vi "MatrixVg_Tdep.vi"(0 "T-table String":string, 3 "Time Stamp":timestamp, 6 "Play Button":bool, 7 "Custom Folder":string, 8 "Settings":T3={"Ring 3"=1, "Ring 2"=4, "Fixed Current mkA"=0.5, "If yes, the current is:"=enum."Radio Selection 1", "Ressitance measurements?"=TRUE, "Commute DC current?"=FALSE} {"Ring 3" items=["1 kOhm", "10 kOhm", "100 kOhm", "1 Mohm", "10 mOhm"]; "Ring 2" items=["1 kOhm", "10 kOhm", "100 kOhm", "1 Mohm", "10 MOhm"]}, 9 "Instruments":T4={"Oscillator"=TRUE, "Addr 1 lock-in"=TRUE, "Addr 1 lock-in oop"=TRUE, "Addr 2 lock-in"=TRUE, "Addr 2 lock-in oop"=TRUE, "Addr 3 lock-in"=FALSE, "Addr 3 lock-in oop"=FALSE, "Voltage (Vk1)"=FALSE, "Current (Ik1)"=TRUE, "Voltage (Vk2)"=FALSE, "Current (Ik2)"=FALSE, "Voltage (Vk3)"=FALSE, "Current (Ik3)"=FALSE, "Channel 1 (Vnano1)  "=FALSE, "Channel 2 (Vnano1b)"=FALSE, "Channel 1 (Vnano2)   "=FALSE, "Channel 2 (Vnano2b)"=FALSE, "Thermometer 1 (T1)"=TRUE, "Magnetic Field (B)"=TRUE, "Capacitance (C) and Loss (L)"=FALSE}, 11 "TCluster":T2={"Starting T (K)"=-1.0, "Final T (K)"=1.0, "Step (T)"=1.0, "Stabillisation, min"=1.0, "Wait 1st point?"=FALSE} {"Final T (K)" min=-4.0 max=4.0 step=0.1 format="%.2f"; "Stabillisation, min" format="%.2f"; "Step (T)" min=0.0 max=1.0 step=0.01 format="%_4f"; "Starting T (K)" min=-4.0 max=4.0 step=0.1 format="%.2f"}) -> ()   [LabVIEW 2017]
uses:
  <vilib>/Utility/file.llb/Read From Spreadsheet File (DBL).vi
panel:
  in  "VgCluster":T1={"V1 (V)"=-1.0, "V2 (V)"=1.0, "Sweep rate, V/min"=1.0, "Time btw \npoints, sec"=1.0, "points at each Vg"=1, "Compliance, mkA"=0.05, "No-record rate, V/min"=30.0, "Full sweep?"=FALSE} {"No-record rate, V/min" min=0.0 max=1.0 step=0.01 format="%_4f"; "V2 (V)" min=-4.0 max=4.0 step=0.1 format="%.2f"; "Compliance, mkA" min=0.0 max=1.0 step=0.01 format="%.3f"; "Time btw \npoints, sec" format="%.2f"; "Sweep rate, V/min" min=0.0 max=1.0 step=0.01 format="%_4f"; "V1 (V)" min=-4.0 max=4.0 step=0.1 format="%.2f"}
  out "Communication":string
  out "T Array":dbl[](array[numeric])
  out "Experiment ends at:":string
  out "Hours":dbl format="%.1f"
  out "Estimated time of experiment:":i16
  out "ArraySens":i8[](array[numeric])
  out "ArrayOsc":dbl[](array[numeric])
  out "# of configurations":i8
  out "Large Array":bool[][][](array[boolean])
  out "Contact configuration file (*.conf)":path
  # "hours"
  # "min.="
  # "Values of T can be also entered as the table by copying\nand pasting a column of numbers in a \"T table\" string at the \nfar right side of this window."
  # "Lock-in Amplifiers"
  # "Temperature"
  # "SourceMeters"
  # "Nanovoltmeters"
  # "Main"
  # "(not recommended, too slow)"
  # "Magnetic Field"
  # "Capacitance & Loss"
  # "(not recommended, too slow)"
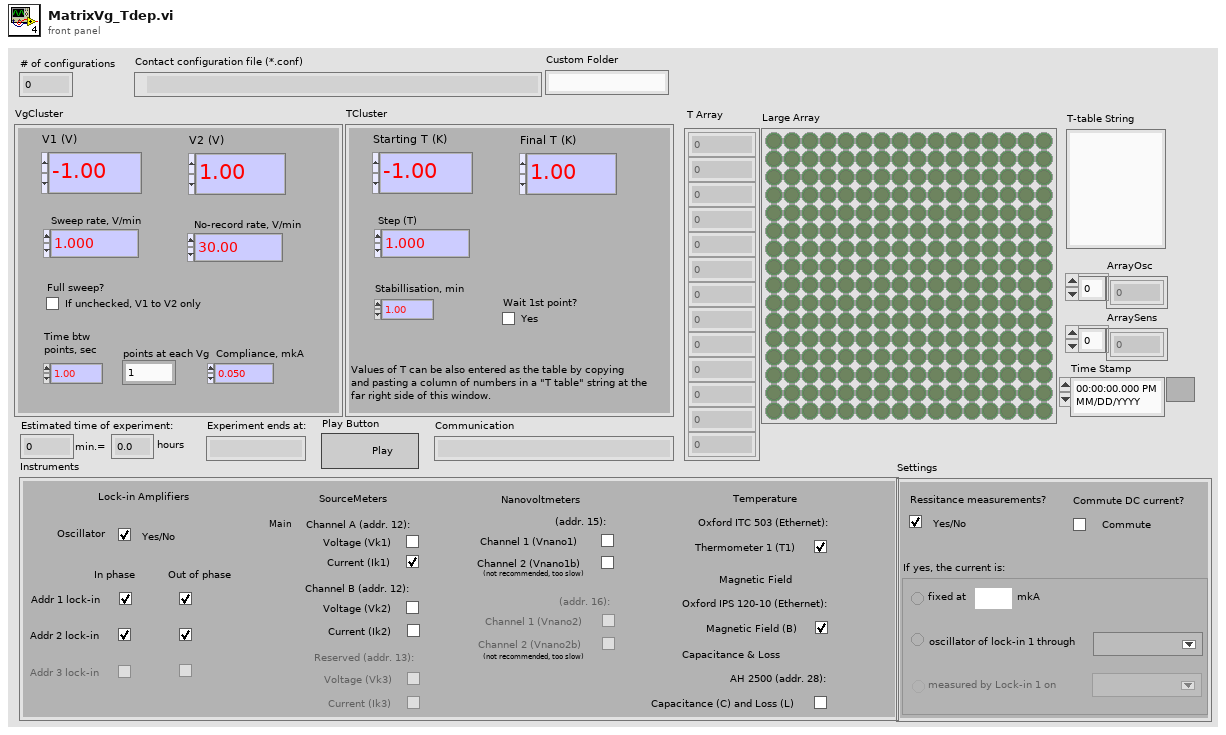
[diagram p1: front panel]
types:
  T1 = cluster{"V1 (V)":dbl, "V2 (V)":dbl, "Sweep rate, V/min":dbl, "Time btw \npoints, sec":dbl, "points at each Vg":i32, "Compliance, mkA":dbl, "No-record rate, V/min":dbl, "Full sweep?":bool}
  T2 = cluster{"Starting T (K)":dbl, "Final T (K)":dbl, "Step (T)":dbl, "Stabillisation, min":dbl, "Wait 1st point?":bool}
  T3 = cluster{"Ring 3":u16, "Ring 2":u16, "Fixed Current mkA":dbl, "If yes, the current is:":enum32{"Radio Selection 1", "Radio Selection 2", "Radio Selection 3"}, "Ressitance measurements?":bool, "Commute DC current?":bool}
  T4 = cluster{"Oscillator":bool, "Addr 1 lock-in":bool, "Addr 1 lock-in oop":bool, "Addr 2 lock-in":bool, "Addr 2 lock-in oop":bool, "Addr 3 lock-in":bool, "Addr 3 lock-in oop":bool, "Voltage (Vk1)":bool, "Current (Ik1)":bool, "Voltage (Vk2)":bool, "Current (Ik2)":bool, "Voltage (Vk3)":bool, "Current (Ik3)":bool, "Channel 1 (Vnano1)  ":bool, "Channel 2 (Vnano1b)":bool, "Channel 1 (Vnano2)   ":bool, "Channel 2 (Vnano2b)":bool, "Thermometer 1 (T1)":bool, "Magnetic Field (B)":bool, "Capacitance (C) and Loss (L)":bool}
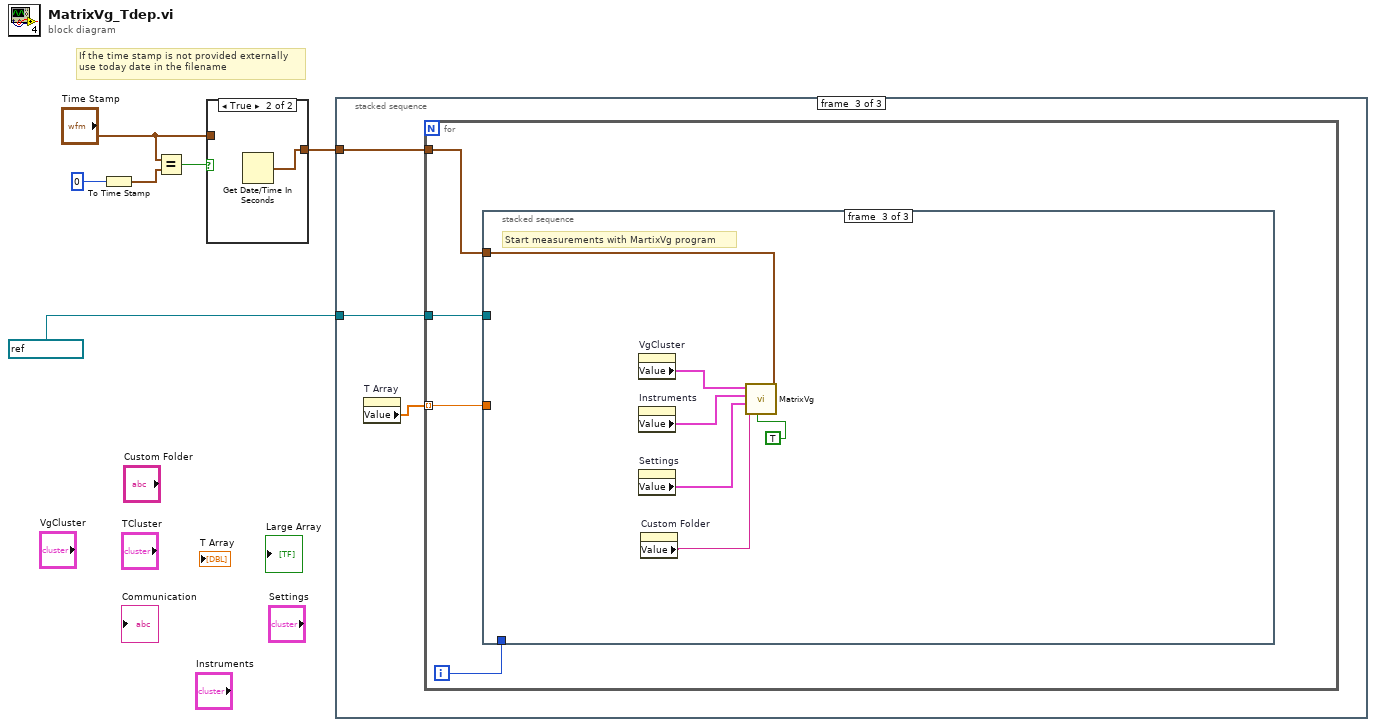
[diagram p0: block diagram]
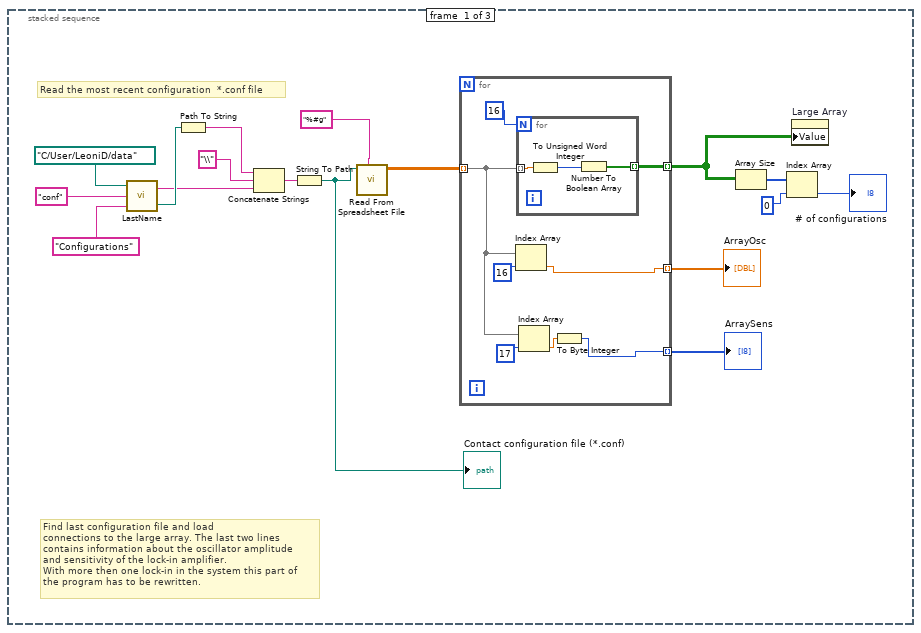
[diagram p3: hidden frame]
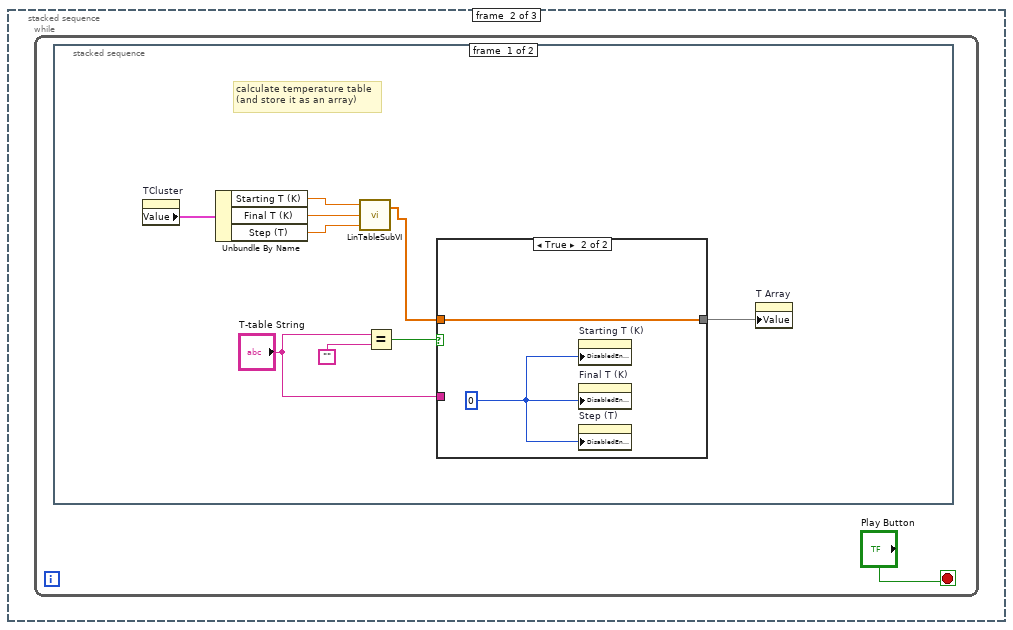
[diagram p4: hidden frame]
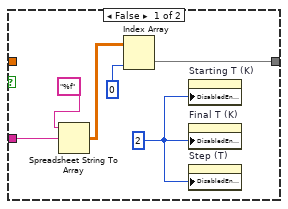
[diagram p5: hidden frame]
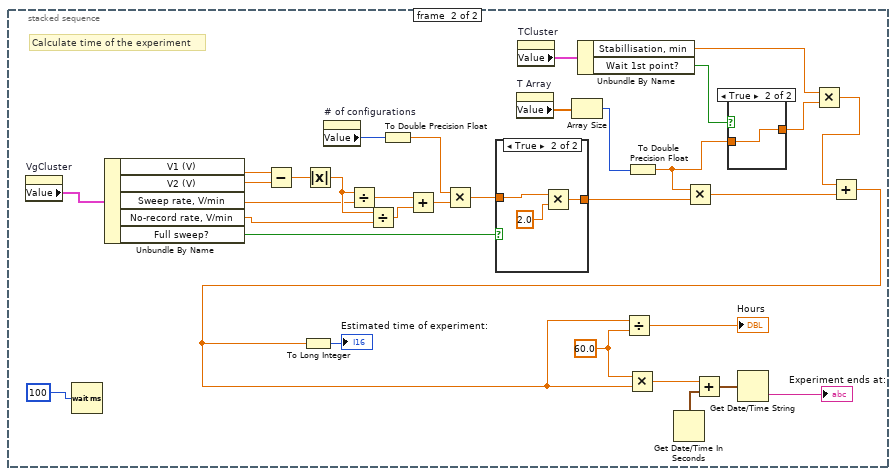
[diagram p6: hidden frame]
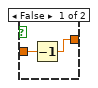
[diagram p7: hidden frame]
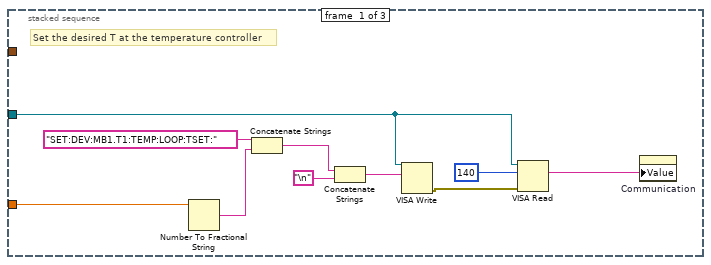
[diagram p9: hidden frame]
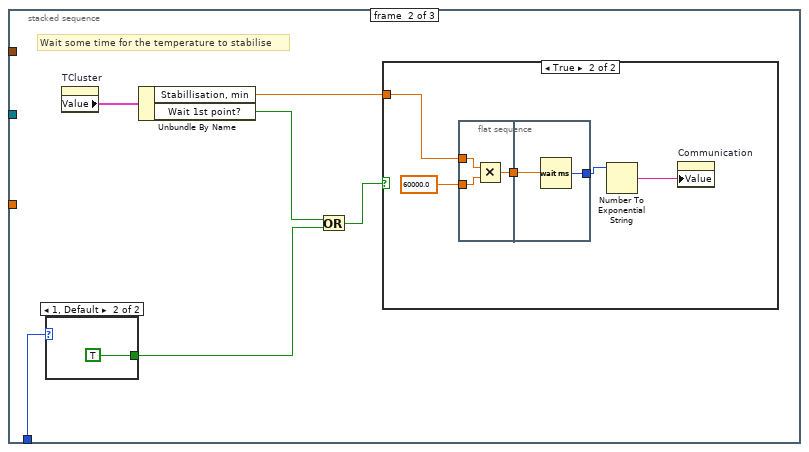
[diagram p10: hidden frame]
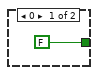
[diagram p12: hidden frame]
diagram:
  # "If the time stamp is not provided externally\nuse today date in the filename"
  n1 = To Time Stamp(1:0) -> (0:w5:timestamp)
  n2 = Equal?(x="Time Stamp", y=w5) -> (x = y?=w4:bool)
  n3 = case shown="True" w4 {
    tunnel: "Time Stamp" -> [w7 _]
    tunnel: [w7 w8] -> w2
    frame False {
    }
    frame True {
      n4 = Get Date/Time In Seconds() -> (seconds since 1Jan1904=w8:timestamp)
    }
  }
  n5 = stacked-sequence {
    tunnel: w2 -> [_ _ w95]
    tunnel: refnum<visa-resource-name> "itcetherT" ("VISA resource name") -> [_ _ w97]
    frame #0 {
      # "Read the most recent configuration  *.conf file"
      # "Find last configuration file and load \nconnections to the large array. The last two lines \ncontains information about the oscillator amplitude\nand sensitivity of the lock-in amplifier.\nWith more then one lock-in in the system this part of \nthe program has to be rewritten."
      n6 = call "LastName.vi"("Custom Folder"="Configurations", "Extention"="conf", "User Data Folder"=path "C:/User/LeoniD/data") -> ("created path"=w21:path, "String"=w20:string)
      n7 = Path To String(path=w21) -> (string=w25:string)
      n8 = Concatenate Strings(w25, "\\", w20) -> (w23:string)
      n9 = String To Path(string=w23) -> (path=w11:path)
      "Contact configuration file (*.conf)" <- w11
      n10 = call-poly <vilib>:"Read From Spreadsheet File.vi"("format (%.3f)"="%#g", "file path (dialog if empty)"=w11) -> ("all rows"=w16:dbl[][])  [unwired: 5 in, 4 out]
      n11 = for {
        tunnel: w16 -> [w29] mode=indexing
        tunnel: [w33] -> w13 mode=indexing
        tunnel: [w28] -> w10 mode=indexing
        tunnel: [w27] -> w9 mode=indexing
        n12 = Index Array(array=w29, index=16) -> (element=w28:dbl)
        n13 = for {
          N: 16 -> [_]
          tunnel: w29 -> [w36] mode=indexing
          tunnel: [w34] -> w33 mode=indexing
          n14 = To Unsigned Word Integer(number=w36) -> (unsigned 16bit integer=w35:u16)
          n15 = Number To Boolean Array(number=w35) -> (Boolean array=w34:bool[])
        }
        n16 = Index Array(array=w29, index=17) -> (element=w30:dbl)
        n17 = To Byte Integer(number=w30) -> (8bit integer=w27:i8)
      }
      "ArrayOsc" <- w10
      "ArraySens" <- w9
      n18 = Array Size(array=w13) -> (size(s)=w15:i32[])
      n19 = Index Array(array=w15, index=0) -> (element=→"# of configurations":i32)
      n20 = property on="Large Array" class="Arr (strict)"("Value"=w13) -> ()  [unwired: 2 in, 2 out]
    }
    frame #1 {
      n21 = while {
        stop <- "Play Button" stop-if-true
        n22 = stacked-sequence {
          frame #0 {
            # "calculate temperature table\n(and store it as an array)"
            n23 = property on="TCluster" class="Clust (strict)"() -> ("Value"=w42:T2)  [unwired: 2 in, 2 out]
            n24 = Unbundle By Name(w42) -> ("Starting T (K)"=w41:dbl, "Final T (K)"=w40:dbl, "Step (T)"=w39:dbl)
            n25 = call "LinTableSubVI.vi"("Step"=w39, "Final"=w40, "Initial"=w41) -> ("Array"=w46:dbl[])  [unwired: 1 in]
            n26 = Equal?(x="T-table String", y="") -> (x = y?=w43:bool)
            n27 = case shown="True" w43 {
              tunnel: [w49 w54] -> w38
              tunnel: w46 -> [_ w54]
              tunnel: "T-table String" -> [w48 _]
              frame False {
                w47 = 2
                n28 = Spreadsheet String To Array(format string="%f", spreadsheet string=w48) -> (array=w51:dbl[][])  [unwired: 2 in]
                n29 = Index Array(array=w51, index (col)=0) -> (element=w49:dbl[])  [unwired: 1 in]
                n30 = property on="Starting T (K)" class="DigNum (strict)"("DisabledEnum"=w47) -> ()  [unwired: 2 in, 2 out]
                n31 = property on="Final T (K)" class="DigNum (strict)"("DisabledEnum"=w47) -> ()  [unwired: 2 in, 2 out]
                n32 = property on="Step (T)" class="DigNum (strict)"("DisabledEnum"=w47) -> ()  [unwired: 2 in, 2 out]
              }
              frame True {
                w53 = 0
                n33 = property on="Starting T (K)" class="DigNum (strict)"("DisabledEnum"=w53) -> ()  [unwired: 2 in, 2 out]
                n34 = property on="Final T (K)" class="DigNum (strict)"("DisabledEnum"=w53) -> ()  [unwired: 2 in, 2 out]
                n35 = property on="Step (T)" class="DigNum (strict)"("DisabledEnum"=w53) -> ()  [unwired: 2 in, 2 out]
              }
            }
            n36 = property on="T Array" class="Arr (strict)"("Value"=w38) -> ()  [unwired: 2 in, 2 out]
          }
          frame #1 {
            w67 = 60.0
            # "Calculate time of the experiment"
            n37 = property on="VgCluster" class="Clust (strict)"() -> ("Value"=w86:T1)  [unwired: 2 in, 2 out]
            n38 = Wait (ms)(milliseconds to wait=100) -> ()  [unwired: 1 out]
            n39 = Unbundle By Name(w86) -> ("V1 (V)"=w85:dbl, "V2 (V)"=w84:dbl, "Sweep rate, V/min"=w81:dbl, "No-record rate, V/min"=w80:dbl, "Full sweep?"=w74:bool)
            n40 = Subtract(x=w85, y=w84) -> (x-y=w83:dbl)
            n41 = Absolute Value(x=w83) -> (abs(x)=w82:dbl)
            n42 = property on="# of configurations" class="DigNum (strict)"() -> ("Value"=w76:i8)  [unwired: 2 in, 2 out]
            n43 = Divide(x=w82, y=w81) -> (x/y=w79:dbl)
            n44 = Divide(x=w82, y=w80) -> (x/y=w78:dbl)
            n45 = To Double Precision Float(number=w76) -> (double precision float=w75:dbl)
            n46 = Add(x=w79, y=w78) -> (x+y=w77:dbl)
            n47 = Multiply(x=w75, y=w77) -> (x*y=w73:dbl)
            n48 = case shown="True" w74 {
              tunnel: w73 -> [w91 w94]
              tunnel: [w91 w92] -> w62
              frame False {
              }
              frame True {
                n49 = Multiply(x=w94, y=2.0) -> (x*y=w92:dbl)
              }
            }
            n50 = property on="T Array" class="Arr (strict)"() -> ("Value"=w65:dbl[])  [unwired: 2 in, 2 out]
            n51 = property on="TCluster" class="Clust (strict)"() -> ("Value"=w64:T2)  [unwired: 2 in, 2 out]
            n52 = Array Size(array=w65) -> (size(s)=w63:i32)
            n53 = Unbundle By Name(w64) -> ("Stabillisation, min"=w59:dbl, "Wait 1st point?"=w61:bool)
            n54 = To Double Precision Float(number=w63) -> (double precision float=w60:dbl)
            n55 = Get Date/Time In Seconds() -> (seconds since 1Jan1904=w71:timestamp)
            n56 = Multiply(x=w60, y=w62) -> (x*y=w57:dbl)
            n57 = case shown="True" w61 {
              tunnel: [w89 w90] -> w58
              tunnel: w60 -> [w88 w90]
              frame False {
                n58 = Decrement(x=w88) -> (x-1=w89:dbl)
              }
              frame True {
              }
            }
            n59 = Multiply(x=w59, y=w58) -> (x*y=w56:dbl)
            n60 = Add(x=w56, y=w57) -> (x+y=w55:dbl)
            n61 = To Long Integer(number=w55) -> (32bit integer=→"Estimated time of experiment:":i32)
            n62 = Divide(x=w55, y=w67) -> (x/y=→"Hours":dbl)
            n63 = Multiply(x=w67, y=w55) -> (x*y=w66:dbl)
            n64 = Add(x=w66, y=w71) -> (x+y=w70:timestamp)
            n65 = Get Date/Time String(seconds (now)=w70) -> (time string=→"Experiment ends at:":string)  [unwired: 2 in, 1 out]
          }
        }
      }
    }
    frame #2 {
      n66 = property on="T Array" class="Arr (strict)"() -> ("Value"=w96:dbl[])  [unwired: 2 in, 2 out]
      n67 = for {
        tunnel: w97 -> [w101]
        tunnel: w96 -> [w100] mode=indexing
        tunnel: w95 -> [w98]
        i -> [w99]
        n68 = stacked-sequence {
          tunnel: w101 -> [w102 _ _]
          tunnel: w100 -> [w103 _ _]
          tunnel: w99 -> [_ w113 _]
          tunnel: w98 -> [_ _ w130]
          frame #0 {
            # "Set the desired T at the temperature controller"
            n69 = Number To Fractional String(number=w103) -> (F-format string=w110:string)  [unwired: 3 in]
            n70 = Concatenate Strings("SET:DEV:MB1.T1:TEMP:LOOP:TSET:" ("string"), w110) -> (w105:string)
            n71 = Concatenate Strings(w105, "\n") -> (w106:string)
            n72 = VISA Write(VISA resource name=w102, write buffer=w106) -> (error out=w109:errorcluster)  [unwired: 1 in, 2 out]
            n73 = VISA Read(VISA resource name=w102, byte count=140, error in (no error)=w109) -> (read buffer=w104:string)  [unwired: 3 out]
            n74 = property on="Communication" class="Str"("Value"=w104) -> ()  [unwired: 2 in, 2 out]
          }
          frame #1 {
            # "Wait some time for the temperature to stabilise"
            n75 = case shown="1, Default" w113 {
              tunnel: [FALSE TRUE] -> w117
              frame 0 {
              }
              frame 1, Default {
              }
            }
            n76 = property on="TCluster" class="Clust (strict)"() -> ("Value"=w115:T2)  [unwired: 2 in, 2 out]
            n77 = Unbundle By Name(w115) -> ("Stabillisation, min"=w112:dbl, "Wait 1st point?"=w114:bool)
            n78 = Or(x=w114, y=w117) -> (x .or. y?=w116:bool)
            n79 = case shown="True" w116 {
              tunnel: w112 -> [_ w121]
              frame False {
              }
              frame True {
                n80 = flat-sequence {
                  tunnel: w121 -> [w125]
                  tunnel: 60000.0 -> [w124]
                  tunnel: [w123] -> w119
                  tunnel: [w127] -> w122
                  tunnel: w119 -> [w126]
                  frame #0 {
                    n81 = Multiply(x=w125, y=w124) -> (x*y=w123:dbl)
                  }
                  frame #1 {
                    n82 = Wait (ms)(milliseconds to wait=w126) -> (millisecond timer value=w127:u32)
                  }
                }
                n83 = Number To Exponential String(number=w122) -> (E-format string=w118:string)  [unwired: 3 in]
                n84 = property on="Communication" class="Str"("Value"=w118) -> ()  [unwired: 2 in, 2 out]
              }
            }
          }
          frame #2 {
            # "Start measurements with MartixVg program"
            n85 = property on="VgCluster" class="Clust (strict)"() -> ("Value"=w131:T1)  [unwired: 2 in, 2 out]
            n86 = property on="Instruments" class="Clust (strict)"() -> ("Value"=w132:T4)  [unwired: 2 in, 2 out]
            n87 = property on="Settings" class="Clust (strict)"() -> ("Value"=w133:T3)  [unwired: 2 in, 2 out]
            n88 = property on="Custom Folder" class="Str"() -> ("Value"=w135:string)  [unwired: 2 in, 2 out]
            n89 = call "MatrixVg.vi"("Time Stamp"=w130, "Play Button"=TRUE, "Custom Folder"=w135, "Settings"=w133, "Instruments"=w132, "VgCluster"=w131) -> ()  [unwired: 6 in]
          }
        }
      }
    }
  }
